vi "getanglefromlidar.vi"(8 "error in (no error)":errorcluster, 11 "VISA resource name":refnum<visa-resource-name>) -> (0 "error constant":errorcluster, 2 "VISA resource name out":refnum<visa-resource-name>, 3 "Distance from Wall":dbl)   [LabVIEW 2017]
doc: "The myRIO Project template acquires acceleration data from the onboard accelerometer and displays the changes of acceleration values in a waveform chart."
uses:
  040-typeDefs/LidarPoint.ctl
panel:
  out "XY Graph 2":cluster{"X":dbl, "Y":dbl}[](graph)
  out "Strength":dbl
  out "XY Graph":cluster{dbl[], dbl[]}[](graph)
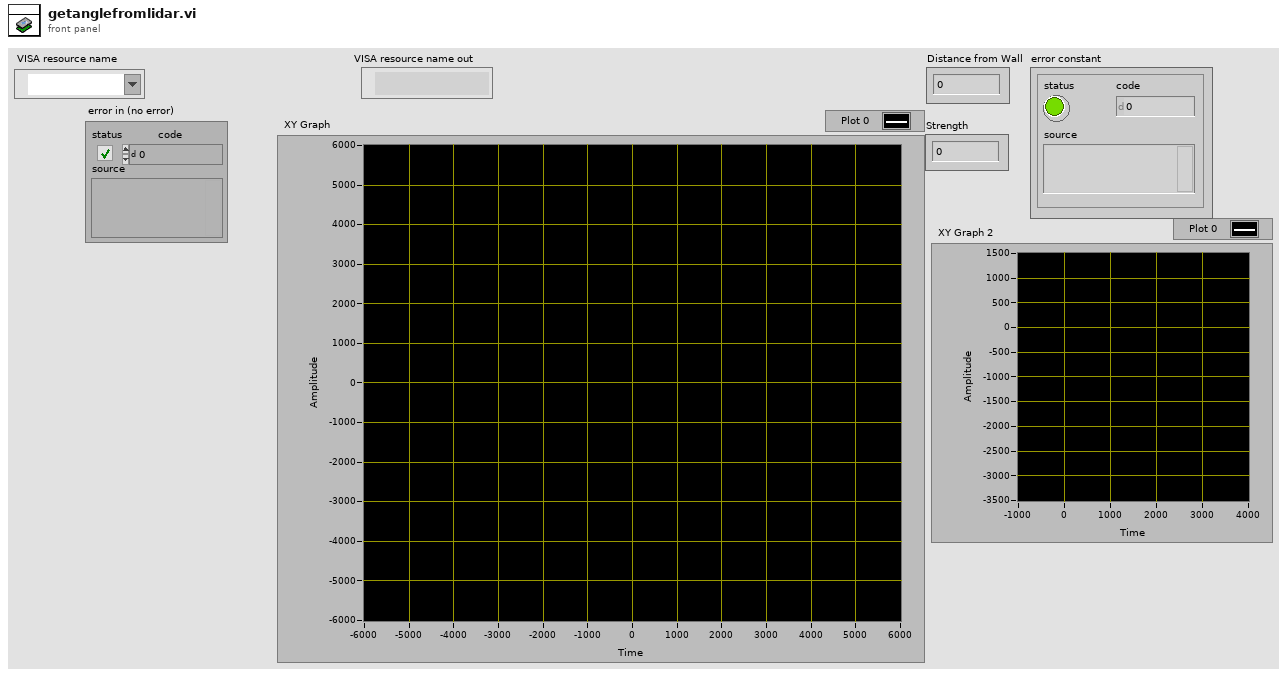
[diagram p1: front panel]
types:
  T1 = typedef "LidarPoint.ctl" = cluster{"X":dbl, "Y":dbl}
  T2 = typedef "XY.ctl" = T1[]
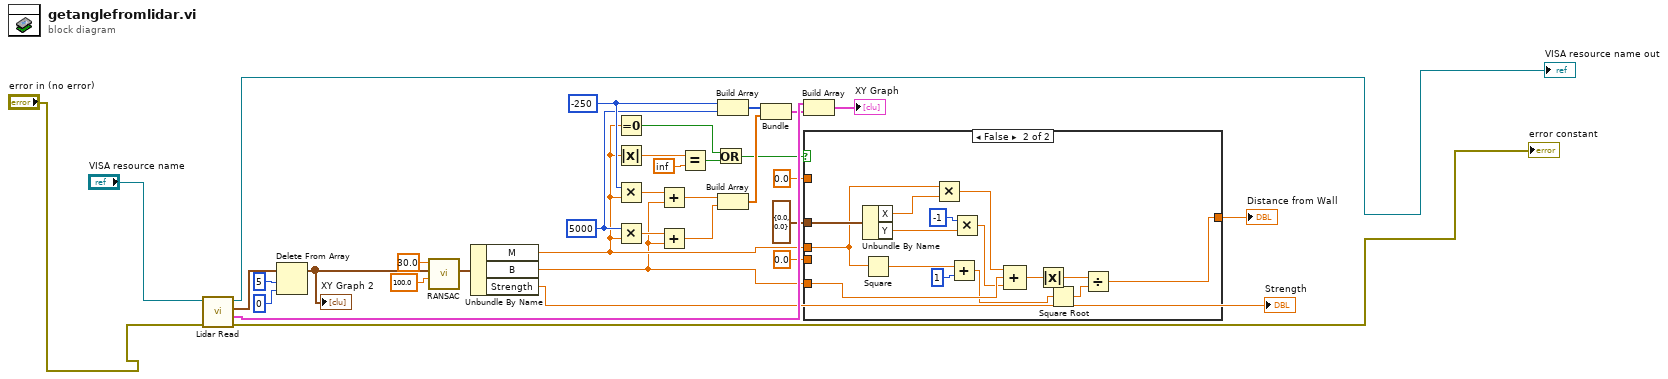
[diagram p0: block diagram]
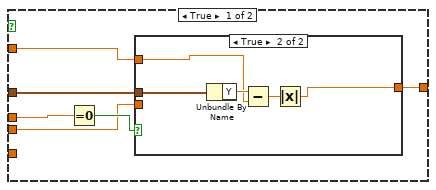
[diagram p2: hidden frame]
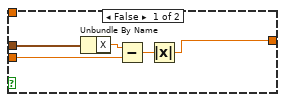
[diagram p3: hidden frame]
diagram:
  w27 = 5000
  w28 = -250
  n1 = call "Lidar Read.vi"("error in (no error)"="error in (no error)", "VISA resource name"="VISA resource name") -> ("error out"=→"error constant":errorcluster, "Visual Out"=w29:cluster{dbl[], dbl[]}, "XY Array"=w19:T2, "VISA resource name out"=→"VISA resource name out":refnum<visa-resource-name>)  [unwired: 5 in]
  n2 = Delete From Array(array=w19, length=5, index=0) -> (array with subset deleted=w16:T2)  [unwired: 1 out]
  "XY Graph 2" <- w16
  n3 = call "RANSAC.vi"("Checks"=100.0, "XY Array"=w16, "Tolerance"=30.0) -> ("Best Line"=w32:cluster{"M":dbl, "B":dbl, "Strength":dbl})  [unwired: 8 in]
  n4 = Unbundle By Name(w32) -> ("M"=w9:dbl, "B"=w8:dbl, "Strength"=→"Strength":dbl)
  n5 = Equal To 0?(x=w9) -> (x = 0?=w12:bool)
  n6 = Absolute Value(x=w9) -> (abs(x)=w14:dbl)
  n7 = Multiply(x=w28, y=w9) -> (x*y=w31:dbl)
  n8 = Multiply(x=w27, y=w9) -> (x*y=w30:dbl)
  n9 = Add(x=w31, y=w8) -> (x+y=w25:dbl)
  n10 = Add(x=w30, y=w8) -> (x+y=w26:dbl)
  n11 = Equal?(x=w14, y=inf) -> (x = y?=w11:bool)
  n12 = Or(x=w12, y=w11) -> (x .or. y?=w10:bool)
  n13 = Build Array(w28, w27) -> (w22:i32[])
  n14 = Build Array(w25, w26) -> (w21:dbl[])
  n15 = Bundle(w22, w21) -> (w24:cluster{i32[], dbl[]})  [unwired: 1 in]
  n16 = Build Array(w29, w24) -> (→"XY Graph":cluster{dbl[], dbl[]}[])
  n17 = case shown="False" w10 {
    tunnel: w8 -> [_ w60]
    tunnel: T1 {"X"=0.0, "Y"=0.0} ("XY") -> [w38 w65]
    tunnel: [w36 w51] -> w5
    tunnel: 0.0 ("X") -> [w37 _]
    tunnel: 0.0 ("Y") -> [w35 _]
    tunnel: w9 -> [w39 w55]
    frame True {
      n18 = Equal To 0?(x=w39) -> (x = 0?=w40:bool)
      n19 = case shown="True" w40 {
        tunnel: w38 -> [w45 w50]
        tunnel: w37 -> [w43 _]
        tunnel: [w41 w46] -> w36
        tunnel: w35 -> [_ w47]
        frame False {
          n20 = Unbundle By Name(w45) -> ("X"=w44:dbl)
          n21 = Subtract(x=w44, y=w43) -> (x-y=w42:dbl)
          n22 = Absolute Value(x=w42) -> (abs(x)=w41:dbl)
        }
        frame True {
          n23 = Unbundle By Name(w50) -> ("Y"=w49:dbl)
          n24 = Subtract(x=w49, y=w47) -> (x-y=w48:dbl)
          n25 = Absolute Value(x=w48) -> (abs(x)=w46:dbl)
        }
      }
    }
    frame False {
      n26 = Unbundle By Name(w65) -> ("X"=w62:dbl, "Y"=w63:dbl)
      n27 = Square(x=w55) -> (x^2=w57:dbl)
      n28 = Multiply(x=w55, y=w62) -> (x*y=w61:dbl)
      n29 = Add(x=w57, y=1) -> (x+y=w52:dbl)
      n30 = Multiply(x=-1, y=w63) -> (x*y=w59:dbl)
      n31 = Compound Arithmetic op=ADD(w61, w60, w59) -> (w58:dbl)
      n32 = Absolute Value(x=w58) -> (abs(x)=w54:dbl)
      n33 = Square Root(x=w52) -> (sqrt(x)=w53:dbl)
      n34 = Divide(x=w54, y=w53) -> (x/y=w51:dbl)
    }
  }
  "Distance from Wall" <- w5
